vi "WLAN_FrequencyOffsetEstimation(LTF).vi"(11 "input cluster":cluster{"t0":dbl, "dt":dbl, "Y":cdb[]}) -> (2 "Frequency offset(LTF)":dbl, 3 "output cluster":cluster{"t0":dbl, "dt":dbl, "Y":cdb[]})   [LabVIEW 2018]
uses:
  <vilib>/Analysis/baseanly.llb/Mean (DBL).vi
  <vilib>/Analysis/NI_AALBase.lvlib
panel:
  out "Waveform Graph 2":dbl[](graph)
  out "Waveform Graph":dbl[](graph)
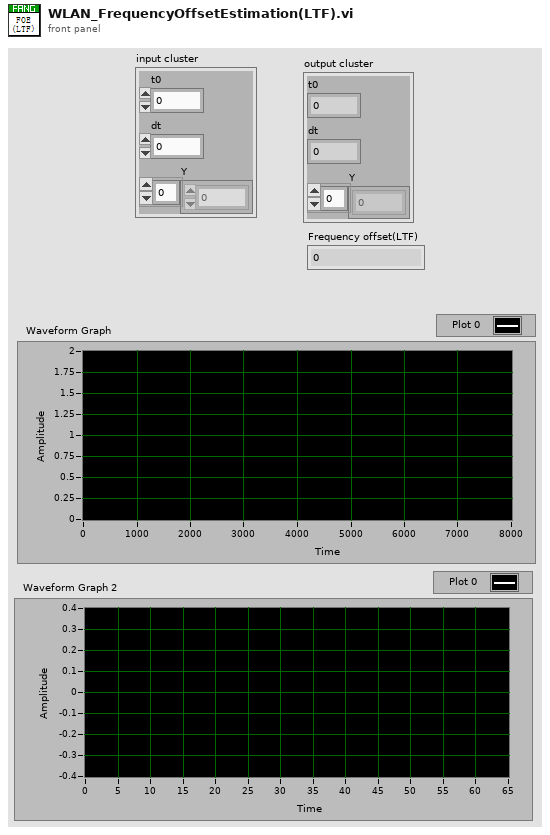
[diagram p1: front panel]
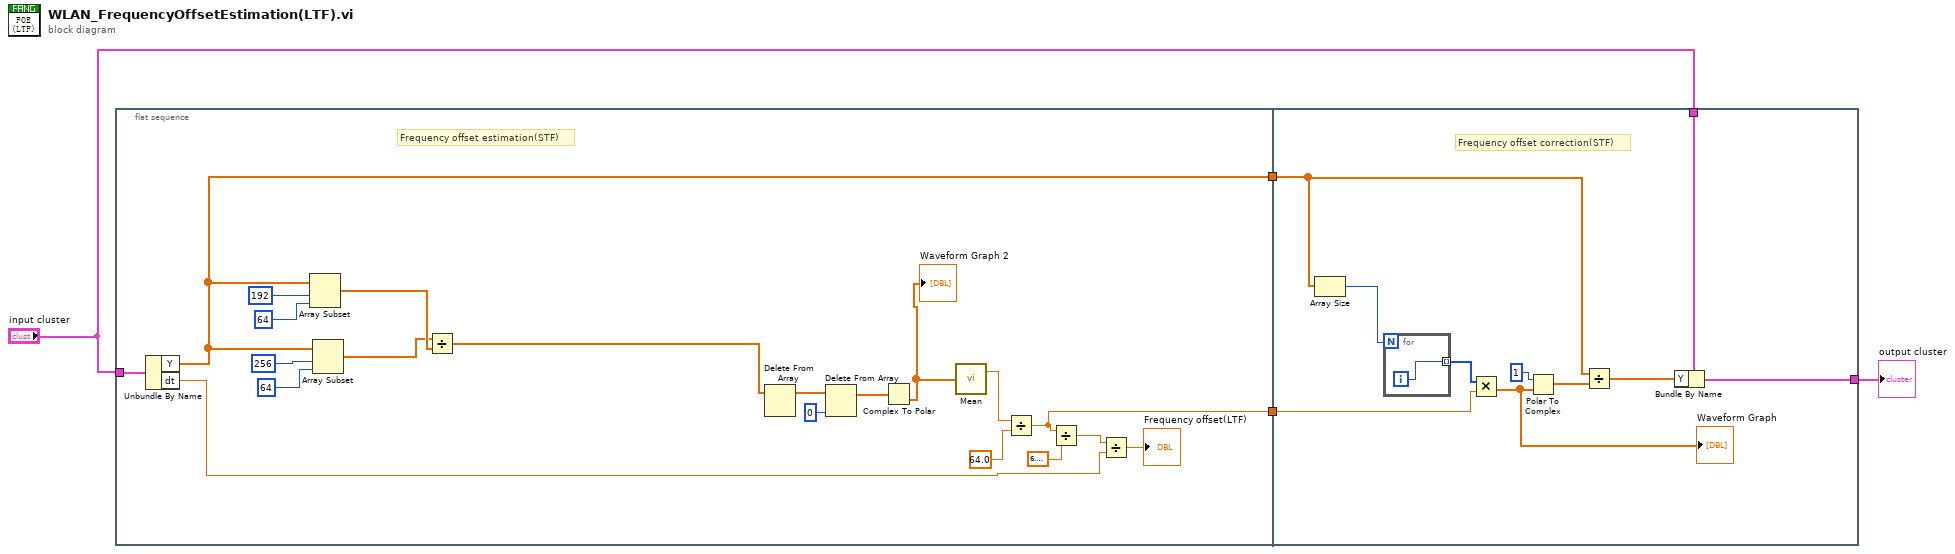
[diagram p0: block diagram]
diagram:
  n1 = flat-sequence {
    tunnel: "input cluster" -> [w18]
    tunnel: [w11] -> w4
    tunnel: [w17] -> w3
    tunnel: w4 -> [w28]
    tunnel: [w25] -> w2
    tunnel: "input cluster" -> [w27]
    tunnel: w3 -> [w26]
    frame #0 {
      # "Frequency offset estimation(STF)"
      n2 = Unbundle By Name(w18) -> ("Y"=w11:cdb[], "dt"=w19:dbl)
      n3 = Array Subset(array=w11, index=192, length=64) -> (w8:cdb[])
      n4 = Array Subset(array=w11, index=256, length=64) -> (w7:cdb[])
      n5 = Divide(x=w7, y=w8) -> (x/y=w9:cdb[])
      n6 = Delete From Array(array=w9) -> (array with subset deleted=w10:cdb[])  [unwired: 2 in, 1 out]
      n7 = Delete From Array(array=w10, index=0) -> (array with subset deleted=w6:cdb[])  [unwired: 1 in, 1 out]
      n8 = Complex To Polar(r * e^(i*theta)=w6) -> (theta=w5:dbl[])  [unwired: 1 out]
      "Waveform Graph 2" <- w5
      n9 = call-poly <vilib>:"Mean.vi"("X"=w5) -> ("mean"=w20:dbl)  [unwired: 1 out]
      n10 = Divide(x=w20, y=64.0) -> (x/y=w17:dbl)
      n11 = Divide(x=w17, y=6.283185307179586) -> (x/y=w22:dbl)
      n12 = Divide(x=w22, y=w19) -> (x/y=→"Frequency offset(LTF)":dbl)
    }
    frame #1 {
      # "Frequency offset correction(STF)"
      n13 = Array Size(array=w28) -> (size(s)=w30:i32)
      n14 = for {
        N: w30 -> [_]
        tunnel: [w35] -> w29 mode=indexing
        i -> [w35]
      }
      n15 = Multiply(x=w29, y=w26) -> (x*y=w34:dbl[])
      "Waveform Graph" <- w34
      n16 = Polar To Complex(1:w34, 2:1) -> (0:w32:cdb[])
      n17 = Divide(x=w28, y=w32) -> (x/y=w33:cdb[])
      n18 = Bundle By Name(cluster=w27, "Y"=w33) -> (w25:cluster{"t0":dbl, "dt":dbl, "Y":cdb[]})
    }
  }
  "output cluster" <- w2
